vi "ZCAN_Transmit_Queue.vi"(0 "devices_handle":u32, 1 "Datas":string, 2 "timeStamp":u64=200, 3 "Chennal":u32, 4 "ID":u32, 5 "error in (no error)":errorcluster caption="错误输入（无错误）", 6 "frame type":T2, 7 "Agreement":T1, 8 "CANFD accelerate":bool, 9 "帧格式":i16) -> (14 "Result":bool, 19 "error out":errorcluster caption="错误输出")   [LabVIEW 2020, in "zlgcan.lvlib"]
uses:
  zlgcan.lvlib
  data_type/ZCANDataObj.ctl
  data_type/canfd_frame.ctl
  data_type/tagZCAN_TransmitFD_Data.ctl
  bin/zlgcan_wrap.dll
  data_type/frame type.ctl
  data_type/Agreement.ctl
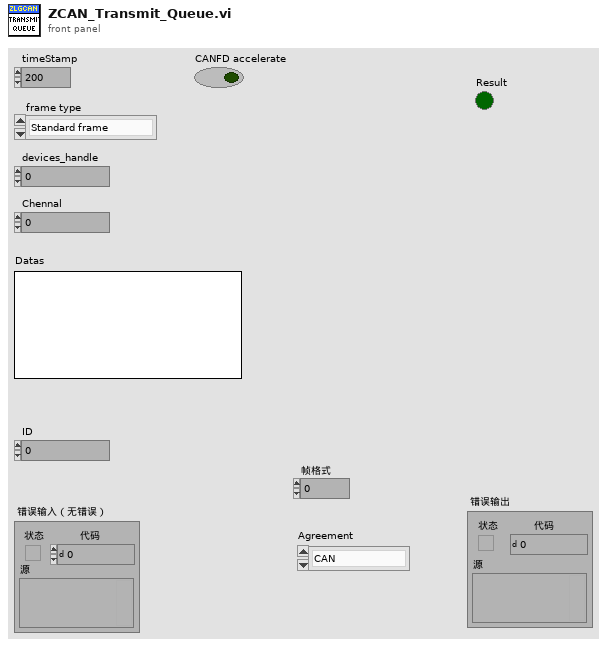
[diagram p1: front panel]
types:
  T1 = typedef "zlgcan.lvlib/Agreement.ctl" = enum16{"CAN", "CANFD"}
  T2 = typedef "zlgcan.lvlib/frame type.ctl" = enum32{"Standard frame", "Extended frame"}
  T3 = typedef "zlgcan.lvlib/tagZCAN_TransmitFD_Data.ctl" = cluster{"canfd_frame":T4, "transmit_type":u32}
  T4 = typedef "zlgcan.lvlib/canfd_frame.ctl" = cluster{"can_id":u32, "len":u8, "flags":u8, "__res0":u8, "__res1":u8, "data":cluster{"CAN数据[0]":u8, "CAN数据[1]":u8, "CAN数据[2]":u8, "CAN数据[3]":u8, "CAN数据[4]":u8, "CAN数据[5]":u8, "CAN数据[6]":u8, "CAN数据[7]":u8, "CAN数据[8]":u8, "CAN数据[9]":u8, "CAN数据[10]":u8, "CAN数据[11] ":u8, "CAN数据[12] ":u8, "CAN数据[13] ":u8, "CAN数据[14] ":u8, "CAN数据[15] ":u8, "CAN数据[16]":u8, "CAN数据[17]":u8, "CAN数据[18]":u8, "CAN数据[19]":u8, "CAN数据[20]":u8, "CAN数据[21]":u8, "CAN数据[22]":u8, "CAN数据[23]":u8, "CAN数据[24] ":u8, "CAN数据[25]":u8, "CAN数据[26]":u8, "CAN数据[27]":u8, "CAN数据[28]":u8, "CAN数据[29]":u8, "CAN数据[30]":u8, "CAN数据[31]":u8, "CAN数据[32]":u8, "CAN数据[33]":u8, "CAN数据[34]":u8, "CAN数据[35]":u8, "CAN数据[36]":u8, "CAN数据[37]":u8, "CAN数据[38]":u8, "CAN数据[39]":u8, "CAN数据[40]":u8, "CAN数据[41]":u8, "CAN数据[42]":u8, "CAN数据[43]":u8, "CAN数据[44]":u8, "CAN数据[45]":u8, "CAN数据[46]":u8, "CAN数据[47]":u8, "CAN数据[48]":u8, "CAN数据[49]":u8, "CAN数据[50]":u8, "CAN数据[51]":u8, "CAN数据[52]":u8, "CAN数据[53]":u8, "CAN数据[54]":u8, "CAN数据[55]":u8, "CAN数据[56]":u8, "CAN数据[57]":u8, "CAN数据[58]":u8, "CAN数据[59]":u8, "CAN数据[60]":u8, "CAN数据[61]":u8, "CAN数据[62]":u8, "CAN数据[63]":u8}}
  T5 = typedef "zlgcan.lvlib/ZCANDataObj.ctl" = cluster{"dataType":u8, "chnl":u8, "flag":cluster{"reserved":u16}, "extraData":cluster{"[0]":u8, "[1]":u8, "[2]":u8, "[3]":u8}, "data":cluster{"canCANFDData":cluster{"timeStamp":u64, "flag":cluster{"unionVal":u32, "rawVal":u32}, "extraData":cluster{"[0]":u8, "[1]":u8, "[2]":u8, "[3]":u8}, "frame":T3}, "raw":cluster{"[0]":u8, "[1]":u8, "[2]":u8, "[3]":u8, "[4]":u8, "[5]":u8, "[6]":u8, "[7]":u8, "[8]":u8, "[9]":u8, "[10]":u8, "[11]":u8, "[12]":u8, "[13]":u8, "[14]":u8, "[15]":u8, "[16]":u8, "[17]":u8, "[18]":u8, "[19]":u8, "[20]":u8, "[21]":u8, "[22]":u8, "[23]":u8, "[24]":u8, "[25]":u8, "[26]":u8, "[27]":u8, "[28]":u8, "[29]":u8, "[30]":u8, "[31]":u8, "[32]":u8, "[33]":u8, "[34]":u8, "[35]":u8, "[36]":u8, "[37]":u8, "[38]":u8, "[39]":u8, "[40]":u8, "[41]":u8, "[42]":u8, "[43]":u8, "[44]":u8, "[45]":u8, "[46]":u8, "[47]":u8, "[48]":u8, "[49]":u8, "[50]":u8, "[51]":u8, "[52]":u8, "[53]":u8, "[54]":u8, "[55]":u8, "[56]":u8, "[57]":u8, "[58]":u8, "[59]":u8, "[60]":u8, "[61]":u8, "[62]":u8, "[63]":u8, "[64]":u8, "[65]":u8, "[73]":u8, "[72]":u8, "[71]":u8, "[70]":u8, "[69]":u8, "[68]":u8, "[67]":u8, "[66]":u8, "[74]":u8, "[75]":u8, "[83]":u8, "[82]":u8, "[81]":u8, "[80]":u8, "[79]":u8, "[78]":u8, "[77]":u8, "[76]":u8, "[84]":u8, "[85]":u8, "[91]":u8, "[90]":u8, "[89]":u8, "[88]":u8, "[87]":u8, "[86]":u8}}}
  T6 = cluster{"Array[0]":u32, "Array[1]":u32, "Array[2]":u32, "Array[3]":u32, "Array[4]":u32, "Array[5]":u32, "Array[6]":u32, "Array[7]":u32, "Array[8]":u32, "Array[9]":u32, "Array[10]":u32, "Array[11]":u32, "Array[12]":u32, "Array[13]":u32, "Array[14]":u32, "Array[15]":u32, "Array[16]":u32, "Array[17]":u32, "Array[18]":u32, "Array[19]":u32, "Array[20]":u32, "Array[21]":u32, "Array[22]":u32, "Array[23]":u32, "Array[24]":u32, "Array[25]":u32, "Array[26]":u32, "Array[27]":u32, "Array[28]":u32, "Array[29]":u32, "Array[30]":u32, "Array[31]":u32, "Array[32]":u32, "Array[33]":u32, "Array[34]":u32, "Array[35]":u32, "Array[36]":u32, "Array[37]":u32, "Array[38]":u32, "Array[39]":u32, "Array[40]":u32, "Array[41]":u32, "Array[42]":u32, "Array[43]":u32, "Array[44]":u32, "Array[45]":u32, "Array[46]":u32, "Array[47]":u32, "Array[48]":u32, "Array[49]":u32, "Array[50]":u32, "Array[51]":u32, "Array[52]":u32, "Array[53]":u32, "Array[54]":u32, "Array[55]":u32, "Array[56]":u32, "Array[57]":u32, "Array[58]":u32, "Array[59]":u32, "Array[60]":u32, "Array[61]":u32, "Array[62]":u32, "Array[63]":u32}
  T7 = cluster{"[0]":u32, "[1]":u32, "[2]":u32, "[3]":u32, "[4]":u32, "[5]":u32, "[6]":u32, "[7]":u32, "[8]":u32, "[9]":u32, "[10]":u32, "[11]":u32, "[12]":u32, "[13]":u32, "[14]":u32, "[15]":u32, "[16]":u32, "[17]":u32, "[18]":u32, "[19]":u32, "[20]":u32, "[21]":u32, "[22]":u32, "[23]":u32, "[24]":u32, "[25]":u32, "[26]":u32, "[27]":u32, "[28]":u32, "[29]":u32, "[30]":u32, "[31]":u32, "[32]":u32, "[33]":u32, "[34]":u32, "[35]":u32, "[36]":u32, "[37]":u32, "[38]":u32, "[39]":u32, "[40]":u32, "[41]":u32, "[42]":u32, "[43]":u32, "[44]":u32, "[45]":u32, "[46]":u32, "[47]":u32, "[48]":u32, "[49]":u32, "[50]":u32, "[51]":u32, "[52]":u32, "[53]":u32, "[54]":u32, "[55]":u32, "[56]":u32, "[57]":u32, "[58]":u32, "[59]":u32, "[60]":u32, "[61]":u32, "[62]":u32, "[63]":u32}
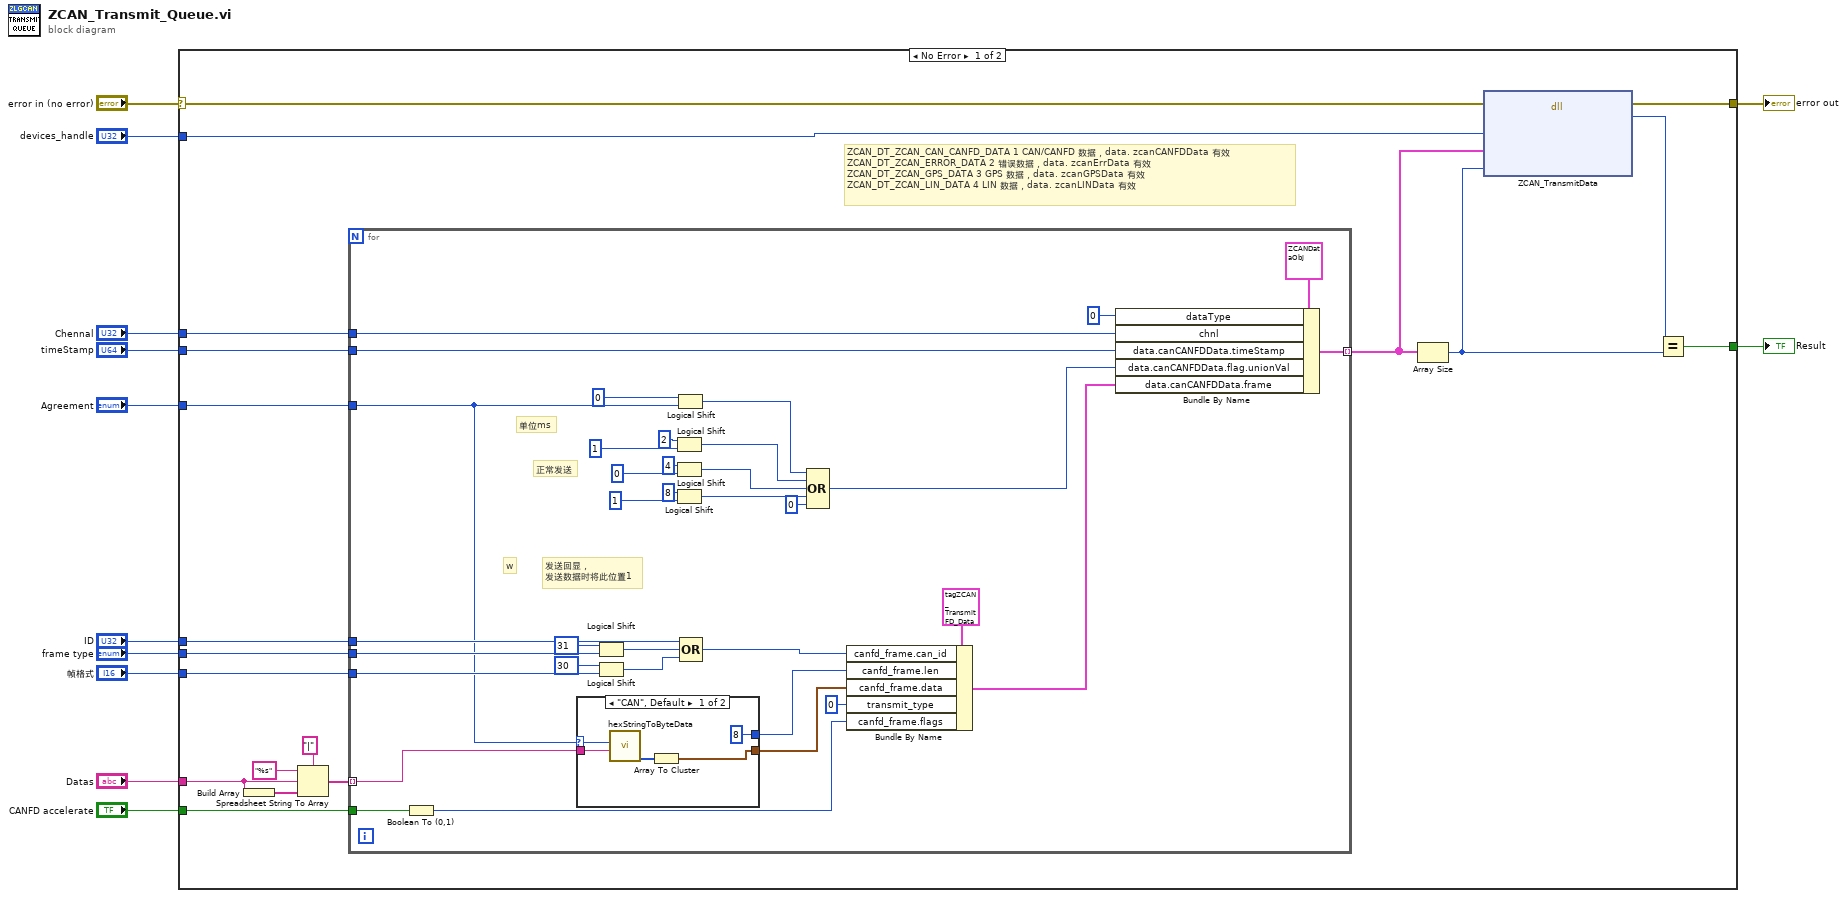
[diagram p0: block diagram]
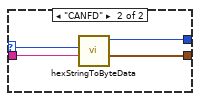
[diagram p2: hidden frame]
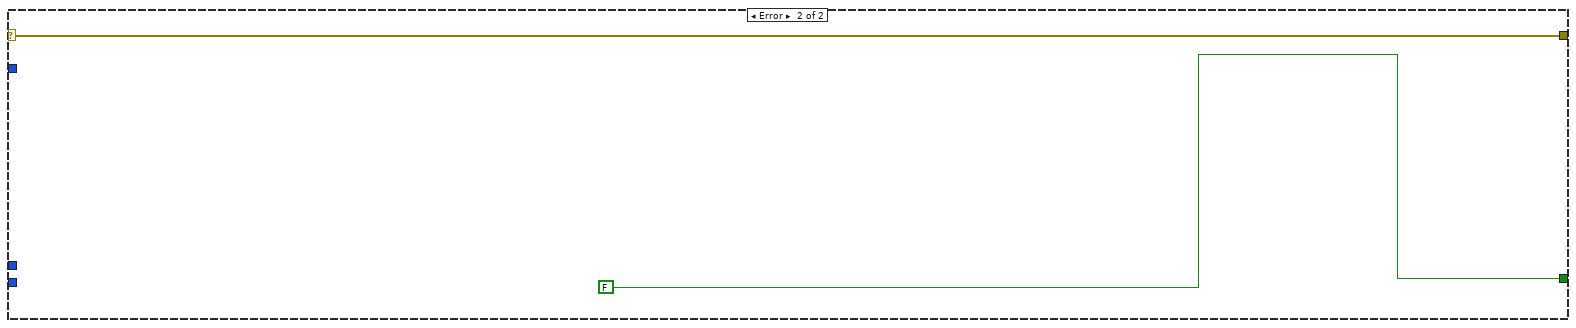
[diagram p3: hidden frame]
diagram:
  n1 = case shown="No Error" "error in (no error)" {
    selector: "error in (no error)" -> [w23 w77]
    tunnel: [w24 w77] -> w12
    tunnel: "devices_handle" -> [w21 _]
    tunnel: "Datas" -> [w26 _]
    tunnel: [w27 FALSE] -> w8
    tunnel: "frame type" -> [w25 _]
    tunnel: "ID" -> [w14 _]
    tunnel: "Agreement" -> [w20 _]
    tunnel: "Chennal" -> [w19 _]
    tunnel: "CANFD accelerate" -> [w18 _]
    tunnel: "帧格式" -> [w15 _]
    tunnel: "timeStamp" -> [w13 _]
    frame No Error {
      # "ZCAN_DT_ZCAN_CAN_CANFD_DATA 1 CAN/CANFD 数据，data. zcanCANFDData 有效\nZCAN_DT_ZCAN_ERROR_DATA 2 错误数据，data. zcanErrData 有效\nZCAN_DT_ZCAN_GPS_DATA 3 GPS 数据，data. zcanGPSData 有效\nZCAN_DT_ZCAN_LIN_DATA 4 LIN 数据，data. zcanLINData 有效"
      n2 = Build Array(w26) -> (w31:string[])
      n3 = Spreadsheet String To Array(delimiter (Tab)="|", format string="%s", spreadsheet string=w26, array type (2D Dbl)=w31) -> (array=w28:string[])
      n4 = for {
        tunnel: w28 -> [w34] mode=indexing
        tunnel: w25 -> [w38]
        tunnel: w20 -> [w35]
        tunnel: w19 -> [w55]
        tunnel: [w54] -> w17 mode=indexing
        tunnel: w18 -> [w52]
        tunnel: w15 -> [w37]
        tunnel: w14 -> [w36]
        tunnel: w13 -> [w49]
        # "w"
        # "发送回显，\n发送数据时将此位置1"
        # "正常发送"
        # "单位ms"
        n5 = Boolean To (0,1)(Boolean=w52) -> (0, 1=w33:i16)
        n6 = case shown="\"CAN\", Default" w35 {
          selector: w35 -> [w71 w73]
          tunnel: [u8 8 ("字节数") w75] -> w42
          tunnel: [w69 w74] -> w40
          tunnel: w34 -> [w67 w72]
          frame "CAN", Default {
            n7 = call "hexStringToByteData.vi"("数据输入"=w67, "协议"=w71) -> ("Array"=w70:u32[])  [unwired: 6 in, 3 out]
            n8 = Array To Cluster(array=w70) -> (cluster=w69:T6)
          }
          frame "CANFD" {
            n9 = call "hexStringToByteData.vi"("数据输入"=w72, "协议"=w73) -> ("CANFD_data"=w74:T7, "字节数"=w75:u8)  [unwired: 6 in, 2 out]
          }
        }
        n10 = Logical Shift(y=i16 31, x=w38) -> (x << y=w47:u32)
        n11 = Logical Shift(y=i16 30, x=w37) -> (x << y=w44:i16)
        n12 = Logical Shift(y=i16 2, x=u32 1 ("y")) -> (x << y=w51:u32)
        n13 = Logical Shift(y=i16 4, x=u32 0 ("y")) -> (x << y=w59:u32)
        n14 = Logical Shift(y=i16 8, x=u32 1 ("y")) -> (x << y=w58:u32)
        n15 = Logical Shift(y=i16 0, x=w35) -> (x << y=w56:u32)
        n16 = Compound Arithmetic op=OR ("复合运算")(w36, w47, w44) -> (w43:u32)
        n17 = Compound Arithmetic op=OR ("复合运算")(w56, w51, w59, w58, u32 0 ("value")) -> (w48:u32)
        n18 = Bundle By Name(cluster=T3 {"canfd_frame"={"can_id"=0, "len"=0, "flags"=0, "__res0"=0, "__res1"=0, "data"={"CAN数据[0]"=0, "CAN数据[1]"=0, "CAN数据[2]"=0, "CAN数据[3]"=0, "CAN数据[4]"=0, "CAN数据[5]"=0, "CAN数据[6]"=0, "CAN数据[7]"=0, "CAN数据[8]"=0, "CAN数据[9]"=0, "CAN数据[10]"=0, "CAN数据[11] "=0, "CAN数据[12] "=0, "CAN数据[13] "=0, "CAN数据[14] "=0, "CAN数据[15] "=0, "CAN数据[16]"=0, "CAN数据[17]"=0, "CAN数据[18]"=0, "CAN数据[19]"=0, "CAN数据[20]"=0, "CAN数据[21]"=0, "CAN数据[22]"=0, "CAN数据[23]"=0, "CAN数据[24] "=0, "CAN数据[25]"=0, "CAN数据[26]"=0, "CAN数据[27]"=0, "CAN数据[28]"=0, "CAN数据[29]"=0, "CAN数据[30]"=0, "CAN数据[31]"=0, "CAN数据[32]"=0, "CAN数据[33]"=0, "CAN数据[34]"=0, "CAN数据[35]"=0, "CAN数据[36]"=0, "CAN数据[37]"=0, "CAN数据[38]"=0, "CAN数据[39]"=0, "CAN数据[40]"=0, "CAN数据[41]"=0, "CAN数据[42]"=0, "CAN数据[43]"=0, "CAN数据[44]"=0, "CAN数据[45]"=0, "CAN数据[46]"=0, "CAN数据[47]"=0, "CAN数据[48]"=0, "CAN数据[49]"=0, "CAN数据[50]"=0, "CAN数据[51]"=0, "CAN数据[52]"=0, "CAN数据[53]"=0, "CAN数据[54]"=0, "CAN数据[55]"=0, "CAN数据[56]"=0, "CAN数据[57]"=0, "CAN数据[58]"=0, "CAN数据[59]"=0, "CAN数据[60]"=0, "CAN数据[61]"=0, "CAN数据[62]"=0, "CAN数据[63]"=0}}, "transmit_type"=0} ("tagZCAN_TransmitFD_Data 2"), "canfd_frame.can_id"=w43, "canfd_frame.len"=w42, "canfd_frame.data"=w40, "transmit_type"=u32 0, "canfd_frame.flags"=w33) -> (w39:T3)
        n19 = Bundle By Name(cluster=T5 {"dataType"=0, "chnl"=0, "flag"={"reserved"=0}, "extraData"={"[0]"=0, "[1]"=0, "[2]"=0, "[3]"=0}, "data"={"canCANFDData"={"timeStamp"=0, "flag"={"unionVal"=0, "rawVal"=0}, "extraData"={"[0]"=0, "[1]"=0, "[2]"=0, "[3]"=0}, "frame"={"canfd_frame"={"can_id"=0, "len"=0, "flags"=0, "__res0"=0, "__res1"=0, "data"={"CAN数据[0]"=0, "CAN数据[1]"=0, "CAN数据[2]"=0, "CAN数据[3]"=0, "CAN数据[4]"=0, "CAN数据[5]"=0, "CAN数据[6]"=0, "CAN数据[7]"=0, "CAN数据[8]"=0, "CAN数据[9]"=0, "CAN数据[10]"=0, "CAN数据[11] "=0, "CAN数据[12] "=0, "CAN数据[13] "=0, "CAN数据[14] "=0, "CAN数据[15] "=0, "CAN数据[16]"=0, "CAN数据[17]"=0, "CAN数据[18]"=0, "CAN数据[19]"=0, "CAN数据[20]"=0, "CAN数据[21]"=0, "CAN数据[22]"=0, "CAN数据[23]"=0, "CAN数据[24] "=0, "CAN数据[25]"=0, "CAN数据[26]"=0, "CAN数据[27]"=0, "CAN数据[28]"=0, "CAN数据[29]"=0, "CAN数据[30]"=0, "CAN数据[31]"=0, "CAN数据[32]"=0, "CAN数据[33]"=0, "CAN数据[34]"=0, "CAN数据[35]"=0, "CAN数据[36]"=0, "CAN数据[37]"=0, "CAN数据[38]"=0, "CAN数据[39]"=0, "CAN数据[40]"=0, "CAN数据[41]"=0, "CAN数据[42]"=0, "CAN数据[43]"=0, "CAN数据[44]"=0, "CAN数据[45]"=0, "CAN数据[46]"=0, "CAN数据[47]"=0, "CAN数据[48]"=0, "CAN数据[49]"=0, "CAN数据[50]"=0, "CAN数据[51]"=0, "CAN数据[52]"=0, "CAN数据[53]"=0, "CAN数据[54]"=0, "CAN数据[55]"=0, "CAN数据[56]"=0, "CAN数据[57]"=0, "CAN数据[58]"=0, "CAN数据[59]"=0, "CAN数据[60]"=0, "CAN数据[61]"=0, "CAN数据[62]"=0, "CAN数据[63]"=0}}, "transmit_type"=0}}, "raw"={"[0]"=0, "[1]"=0, "[2]"=0, "[3]"=0, "[4]"=0, "[5]"=0, "[6]"=0, "[7]"=0, "[8]"=0, "[9]"=0, "[10]"=0, "[11]"=0, "[12]"=0, "[13]"=0, "[14]"=0, "[15]"=0, "[16]"=0, "[17]"=0, "[18]"=0, "[19]"=0, "[20]"=0, "[21]"=0, "[22]"=0, "[23]"=0, "[24]"=0, "[25]"=0, "[26]"=0, "[27]"=0, "[28]"=0, "[29]"=0, "[30]"=0, "[31]"=0, "[32]"=0, "[33]"=0, "[34]"=0, "[35]"=0, "[36]"=0, "[37]"=0, "[38]"=0, "[39]"=0, "[40]"=0, "[41]"=0, "[42]"=0, "[43]"=0, "[44]"=0, "[45]"=0, "[46]"=0, "[47]"=0, "[48]"=0, "[49]"=0, "[50]"=0, "[51]"=0, "[52]"=0, "[53]"=0, "[54]"=0, "[55]"=0, "[56]"=0, "[57]"=0, "[58]"=0, "[59]"=0, "[60]"=0, "[61]"=0, "[62]"=0, "[63]"=0, "[64]"=0, "[65]"=0, "[73]"=0, "[72]"=0, "[71]"=0, "[70]"=0, "[69]"=0, "[68]"=0, "[67]"=0, "[66]"=0, "[74]"=0, "[75]"=0, "[83]"=0, "[82]"=0, "[81]"=0, "[80]"=0, "[79]"=0, "[78]"=0, "[77]"=0, "[76]"=0, "[84]"=0, "[85]"=0, "[91]"=0, "[90]"=0, "[89]"=0, "[88]"=0, "[87]"=0, "[86]"=0}}} ("ZCANDataObj"), "dataType"=u8 0 ("Data_Type"), "chnl"=w55, "data.canCANFDData.timeStamp"=w49, "data.canCANFDData.flag.unionVal"=w48, "data.canCANFDData.frame"=w39) -> (w54:T5)
      }
      n20 = Array Size(array=w17) -> (size(s)=w16:i32)
      n21 = dll-call lib="D:/Git/ZLG_USBCANFD/bin/zlgcan_wrap.dll" fn="ZCAN_TransmitData"(error in=w23, "通道句柄"=w21, "数据帧数组"=w17, "数据帧数"=w16) -> (error out=w24:errorcluster, "返回类型"=w22:u32)  [unwired: 5 in, 1 out]
      n22 = Equal?(x=w22, y=w16) -> (x = y?=w27:bool)
    }
    frame Error {
    }
  }
  "error out" <- w12
  "Result" <- w8
